vi "m300pmReport.vi"() -> ()   [LabVIEW 2012]
uses:
  <vilib>/addons/database/Auxilliary.llb/DB Tools Cursor Type.ctl
  <vilib>/Utility/NIReport.llb/NI_report.lvclass
  <vilib>/addons/database/Connection.llb/DB Tools Open Connec (Path).vi
  <vilib>/addons/database/Connection.llb/Conn Execute.vi
  <vilib>/addons/database/Recordset.llb/Rec Fetch Recordset Data (R).vi
  <vilib>/addons/database/Recordset.llb/Rec Destroy - Connection.vi
  <vilib>/Utility/NIReport.llb/Append Text Table to Report (wrap).vi
  <vilib>/addons/database/_DB Variant To Data/Database Variant To Data.xnode
  <vilib>/addons/database/NI_Database_API.lvlib
  <vilib>/Utility/NIReport.llb/Excel/NI_Excel.lvclass
  <vilib>/addons/_office/NI_ReportGenerationToolkit.lvlib
  <vilib>/Utility/SMTP/NI_SMTPEmail.lvlib
panel:
  out "error out 2":errorcluster
  out "concatenated string 2":string
  out "error out 4":errorcluster
  in  "MIME content-type (application/octet-stream)":string="application/octet-stream"
  out "error out 3":errorcluster
  out "concatenated string":string
  in  "transposed array":string[][](array[string])
  out "error out":errorcluster
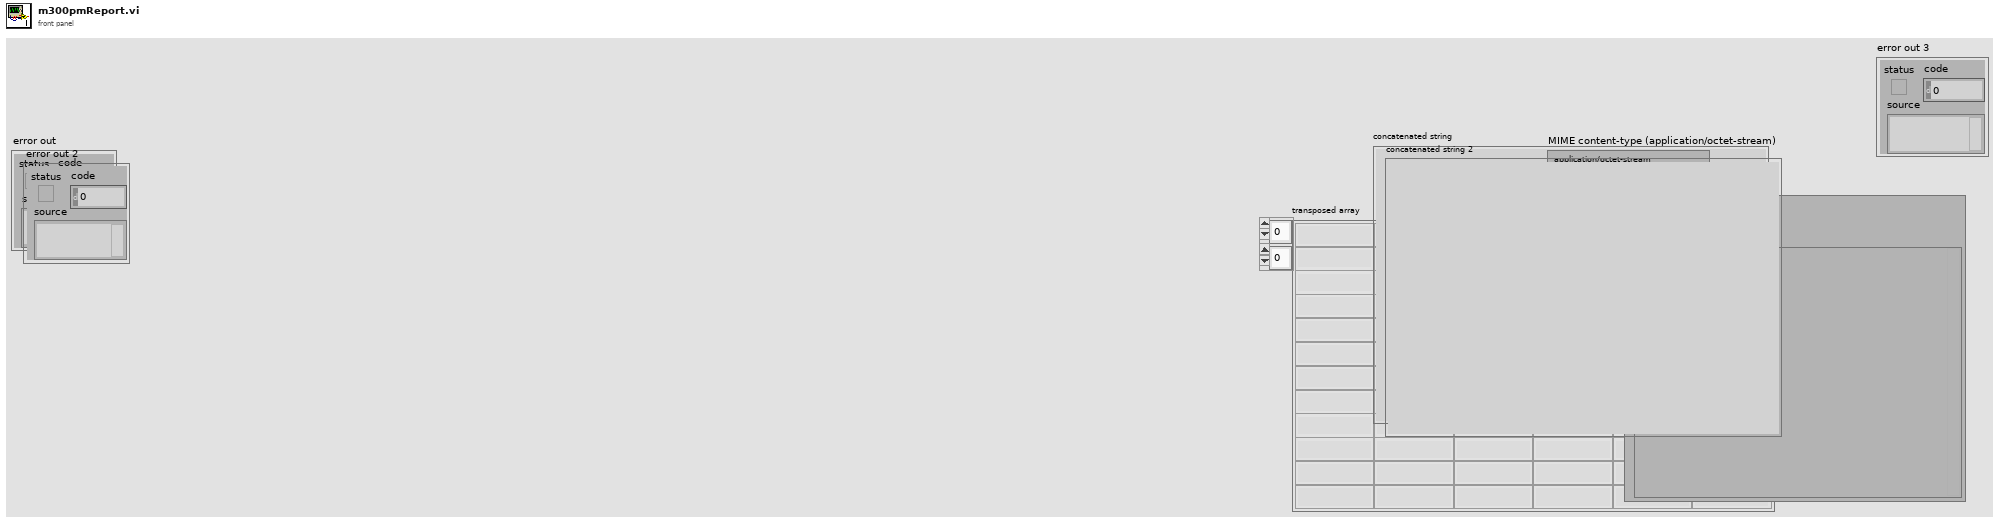
[diagram p1: front panel]
types:
  T1 = enum16{"Standard Report", "HTML", "Word", "Excel"}
  T2 = typedef "NI_Database_API.lvlib/DB Tools Cursor Type.ctl" = enum16{"forward-only", "keyset", "dynamic", "static"}
  T3 = typedef "NI_Database_API.lvlib/Conn ObjectReference.ctl" = refnum<k1>
  T4 = typedef "NI_Database_API.lvlib/Rec ObjectReference.ctl" = refnum<k1>
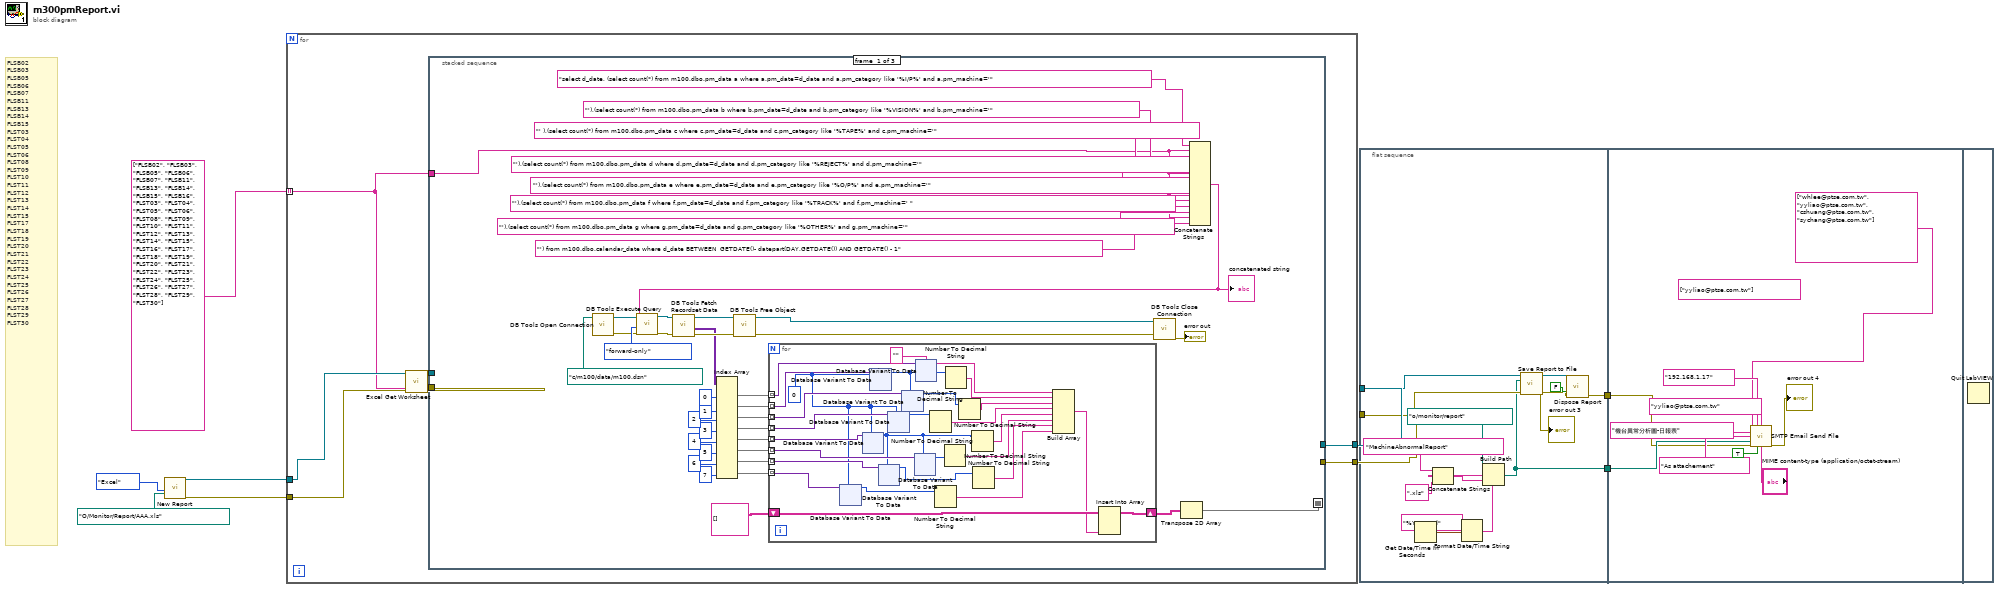
[diagram p0: block diagram]
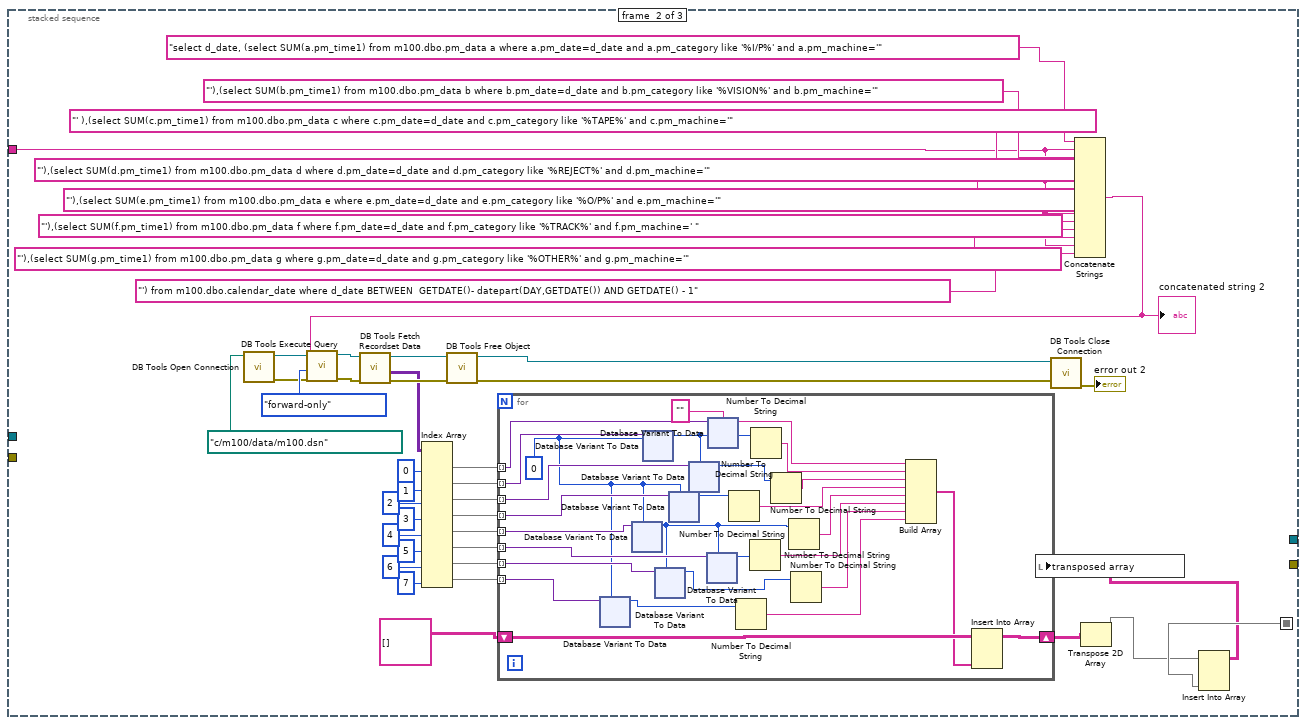
[diagram p2: hidden frame]
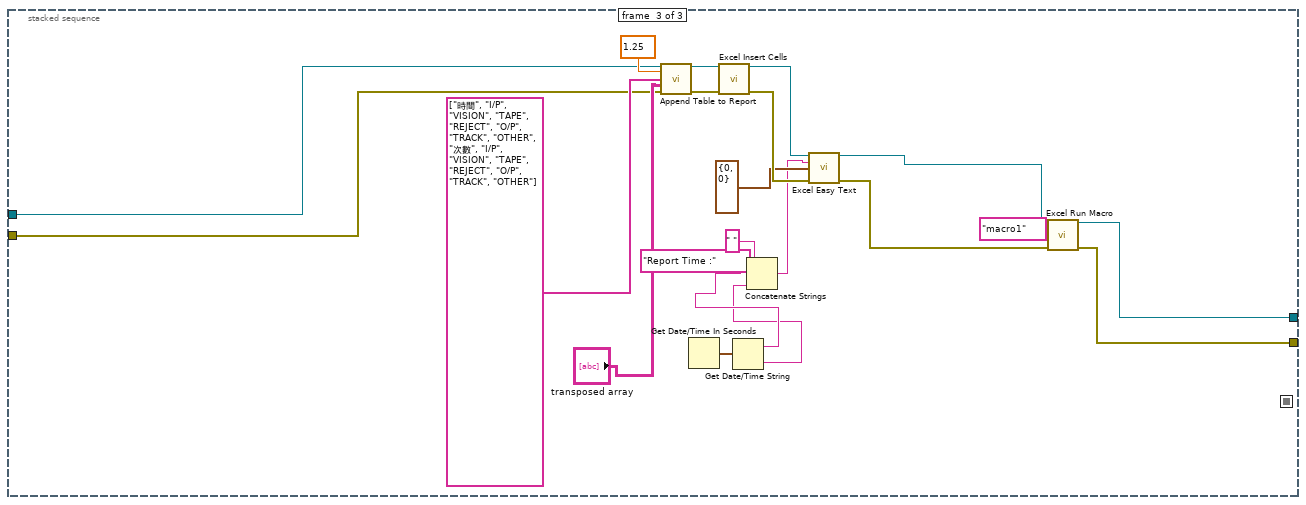
[diagram p3: hidden frame]
diagram:
  # "FLSB02    \nFLSB03    \nFLSB05    \nFLSB06    \nFLSB07    \nFLSB11    \nFLSB13    \nFLSB14    \nFLSB15    \nFLST03    \nFLST04    \nFLST05    \nFLST06    \nFLST08    \nFLST09    \nFLST10    \nFLST11    \nFLST12    \nFLST13    \nFLST14    \nFLST15    \nFLST17    \nFLST18    \nFLST19    \nFLST20    \nFLST21    \nFLST22    \nFLST23    \nFLST24    \nFLST25    \nFLST26    \nFLST27    \nFLST28    \nFLST29    \nFLST30"
  n1 = call <vilib>:"New Report.vi"("report type"=T1."Excel" ("Report Type"), "template (empty)"=path "O:/Monitor/Report/AAA.xls") -> ("report out"=w7:refnum<class "NI_report.lvclass">, "error out"=w6:errorcluster)  [unwired: 12 in]
  n2 = for {
    tunnel: w7 -> [w16]
    tunnel: w6 -> [w15]
    tunnel: string[] ["FLSB02", "FLSB03", "FLSB05", "FLSB06", "FLSB07", "FLSB11", "FLSB13", "FLSB14", "FLSB15", "FLSB16", "FLST03", "FLST04", "FLST05", "FLST06", "FLST08", "FLST09", "FLST10", "FLST11", "FLST12", "FLST13", "FLST14", "FLST15", "FLST16", "FLST17", "FLST18", "FLST19", "FLST20", "FLST21", "FLST22", "FLST23", "FLST24", "FLST25", "FLST26", "FLST27", "FLST28", "FLST29", "FLST30"] -> [w12] mode=indexing
    tunnel: [w11] -> w2
    tunnel: [w10] -> w1
    n3 = call <vilib>:"Excel Get Worksheet.vi"("report in"=w16, "error in (no error)"=w15, "name (\"\")"=w12) -> ("report out"=w14:refnum<class "NI_report.lvclass">, "error out"=w13:errorcluster)  [unwired: 11 in]
    n4 = stacked-sequence {
      seq-local: [w28 _ _] -> [_ w354 _]
      tunnel: w14 -> [_ _ w675]
      tunnel: w13 -> [_ _ w674]
      tunnel: w12 -> [w17 w342 _]
      tunnel: [_ _ w672] -> w11
      tunnel: [_ _ w671] -> w10
      frame #0 {
        n5 = call-poly <vilib>:"DB Tools Open Connection.vi"("connection information"=path "c:/m100/data/m100.dsn") -> ("error out"=w30:errorcluster, "connection reference"=w29:T3)  [unwired: 7 in]
        n6 = Concatenate Strings("select d_date, (select count(*) from m100.dbo.pm_data a where a.pm_date=d_date and a.pm_category like '%I/P%' and a.pm_machine='" ("SQL query"), w17, "'),(select count(*) from m100.dbo.pm_data b where b.pm_date=d_date and b.pm_category like '%VISION%' and b.pm_machine='" ("string"), w17, "' ),(select count(*) from m100.dbo.pm_data c where c.pm_date=d_date and c.pm_category like '%TAPE%' and c.pm_machine='" ("string"), w17, "'),(select count(*) from m100.dbo.pm_data d where d.pm_date=d_date and d.pm_category like '%REJECT%' and d.pm_machine='" ("string"), w17, "'),(select count(*) from m100.dbo.pm_data e where e.pm_date=d_date and e.pm_category like '%O/P%' and e.pm_machine='" ("string"), w17, "'),(select count(*) from m100.dbo.pm_data f where f.pm_date=d_date and f.pm_category like '%TRACK%' and f.pm_machine=' " ("string"), w17, "'),(select count(*) from m100.dbo.pm_data g where g.pm_date=d_date and g.pm_category like '%OTHER%' and g.pm_machine='" ("string"), w17, "') from m100.dbo.calendar_date where d_date BETWEEN  GETDATE()- datepart(DAY,GETDATE()) AND GETDATE() - 1" ("string")) -> (w18:string)
        "concatenated string" <- w18
        n7 = call-poly <vilib>:"DB Tools Execute Query.vi"("error in (no error)"=w30, "cursor type"=DB_Tools_Cursor_Type."forward-only", "SQL query"=w18, "connection reference"=w29) -> ("error out"=w51:errorcluster, "recordset reference"=w53:T4)  [unwired: 4 in]
        n8 = call-poly <vilib>:"DB Tools Fetch Recordset Data.vi"("error in (no error)"=w51, "recordset reference"=w53) -> ("error out"=w50:errorcluster, "recordset data"=w48:variant[][], "recordset reference out"=w52:T4)  [unwired: 3 in]
        n9 = Index Array(array=w48, index (col) #1=0 ("disabled index (col)"), index (col) #2=1 ("index (col)"), index (col) #3=2 ("index (col)"), index (col) #4=3 ("index (col)"), index (col) #5=4 ("index (col)"), index (col) #6=5 ("index (col)"), index (col) #7=6 ("index (col)"), index (col) #8=7 ("index (col)")) -> (element #1=w45:variant[], element #2=w44:variant[], element #3=w36:variant[], element #4=w35:variant[], element #5=w34:variant[], element #6=w33:variant[], element #7=w32:variant[], element #8=w31:variant[])  [unwired: 8 in]
        n10 = call-poly <vilib>:"DB Tools Free Object.vi"("error in (no error)"=w50, "recordset reference"=w52) -> ("error out"=w54:errorcluster, "connection reference"=w55:T3)  [unwired: 8 in]
        n11 = for {
          tunnel: w45 -> [w84] mode=indexing
          tunnel: w44 -> [w85] mode=indexing
          shift-right: [w80] -> w27
          shift-left: string[][] [] ("array") -> [w79]
          tunnel: w36 -> [w77] mode=indexing
          tunnel: w35 -> [w76] mode=indexing
          tunnel: w34 -> [w75] mode=indexing
          tunnel: w33 -> [w74] mode=indexing
          tunnel: w32 -> [w71] mode=indexing
          tunnel: w31 -> [w68] mode=indexing
          w67 = 0
          n12 = xnode "Database Variant To Data"("database variant"=w68, "type"=w67) -> ("data"=w66:i32)  [unwired: 1 in, 1 out]
          n13 = xnode "Database Variant To Data"("database variant"=w75, "type"=w67) -> ("data"=w69:i32)  [unwired: 1 in, 1 out]
          n14 = xnode "Database Variant To Data"("database variant"=w85, "type"=w67) -> ("data"=w65:i32)  [unwired: 1 in, 1 out]
          n15 = xnode "Database Variant To Data"("database variant"=w71, "type"=w69) -> ("data"=w70:i32)  [unwired: 1 in, 1 out]
          n16 = xnode "Database Variant To Data"("database variant"=w76, "type"=w67) -> ("data"=w73:i32)  [unwired: 1 in, 1 out]
          n17 = xnode "Database Variant To Data"("database variant"=w77, "type"=w65) -> ("data"=w64:i32)  [unwired: 1 in, 1 out]
          n18 = xnode "Database Variant To Data"("database variant"=w74, "type"=w69) -> ("data"=w72:i32)  [unwired: 1 in, 1 out]
          n19 = xnode "Database Variant To Data"("database variant"=w84, "type"="") -> ("data"=w82:string)  [unwired: 1 in, 1 out]
          n20 = Number To Decimal String(number=w73) -> (decimal integer string=w59:string)  [unwired: 1 in]
          n21 = Number To Decimal String(number=w66) -> (decimal integer string=w63:string)  [unwired: 1 in]
          n22 = Number To Decimal String(number=w72) -> (decimal integer string=w61:string)  [unwired: 1 in]
          n23 = Number To Decimal String(number=w65) -> (decimal integer string=w81:string)  [unwired: 1 in]
          n24 = Number To Decimal String(number=w64) -> (decimal integer string=w58:string)  [unwired: 1 in]
          n25 = Number To Decimal String(number=w69) -> (decimal integer string=w60:string)  [unwired: 1 in]
          n26 = Number To Decimal String(number=w70) -> (decimal integer string=w62:string)  [unwired: 1 in]
          n27 = Build Array(w82, w81, w58, w59, w60, w61, w62, w63) -> (w78:string[])
          n28 = Insert Into Array(array=w79, new element=w78) -> (w80:string[][])  [unwired: 2 in]
        }
        n29 = call <vilib>:"DB Tools Close Connection.vi"("error in (no error)"=w54, "connection reference"=w55) -> ("error out"=→"error out":errorcluster)  [unwired: 5 in]
        n30 = Transpose 2D Array(2D array=w27) -> (transposed array=w28:string[][])
      }
      frame #1 {
        n31 = call-poly <vilib>:"DB Tools Open Connection.vi"("connection information"=path "c:/m100/data/m100.dsn") -> ("error out"=w358:errorcluster, "connection reference"=w357:T3)  [unwired: 7 in]
        n32 = Concatenate Strings("select d_date, (select SUM(a.pm_time1) from m100.dbo.pm_data a where a.pm_date=d_date and a.pm_category like '%I/P%' and a.pm_machine='" ("SQL query"), w342, "'),(select SUM(b.pm_time1) from m100.dbo.pm_data b where b.pm_date=d_date and b.pm_category like '%VISION%' and b.pm_machine='" ("string"), w342, "' ),(select SUM(c.pm_time1) from m100.dbo.pm_data c where c.pm_date=d_date and c.pm_category like '%TAPE%' and c.pm_machine='" ("string"), w342, "'),(select SUM(d.pm_time1) from m100.dbo.pm_data d where d.pm_date=d_date and d.pm_category like '%REJECT%' and d.pm_machine='" ("string"), w342, "'),(select SUM(e.pm_time1) from m100.dbo.pm_data e where e.pm_date=d_date and e.pm_category like '%O/P%' and e.pm_machine='" ("string"), w342, "'),(select SUM(f.pm_time1) from m100.dbo.pm_data f where f.pm_date=d_date and f.pm_category like '%TRACK%' and f.pm_machine=' " ("string"), w342, "'),(select SUM(g.pm_time1) from m100.dbo.pm_data g where g.pm_date=d_date and g.pm_category like '%OTHER%' and g.pm_machine='" ("string"), w342, "') from m100.dbo.calendar_date where d_date BETWEEN  GETDATE()- datepart(DAY,GETDATE()) AND GETDATE() - 1" ("string")) -> (w343:string)
        "concatenated string 2" <- w343
        n33 = call-poly <vilib>:"DB Tools Execute Query.vi"("error in (no error)"=w358, "cursor type"=DB_Tools_Cursor_Type."forward-only", "SQL query"=w343, "connection reference"=w357) -> ("error out"=w378:errorcluster, "recordset reference"=w380:T4)  [unwired: 4 in]
        n34 = call-poly <vilib>:"DB Tools Fetch Recordset Data.vi"("error in (no error)"=w378, "recordset reference"=w380) -> ("error out"=w377:errorcluster, "recordset data"=w375:variant[][], "recordset reference out"=w379:T4)  [unwired: 3 in]
        n35 = Index Array(array=w375, index (col) #1=0 ("disabled index (col)"), index (col) #2=1 ("index (col)"), index (col) #3=2 ("index (col)"), index (col) #4=3 ("index (col)"), index (col) #5=4 ("index (col)"), index (col) #6=5 ("index (col)"), index (col) #7=6 ("index (col)"), index (col) #8=7 ("index (col)")) -> (element #1=w372:variant[], element #2=w371:variant[], element #3=w364:variant[], element #4=w363:variant[], element #5=w362:variant[], element #6=w361:variant[], element #7=w360:variant[], element #8=w359:variant[])  [unwired: 8 in]
        n36 = call-poly <vilib>:"DB Tools Free Object.vi"("error in (no error)"=w377, "recordset reference"=w379) -> ("error out"=w381:errorcluster, "connection reference"=w382:T3)  [unwired: 8 in]
        n37 = for {
          tunnel: w372 -> [w411] mode=indexing
          tunnel: w371 -> [w412] mode=indexing
          shift-right: [w407] -> w356
          shift-left: string[][] [] ("array") -> [w406]
          tunnel: w364 -> [w404] mode=indexing
          tunnel: w363 -> [w403] mode=indexing
          tunnel: w362 -> [w402] mode=indexing
          tunnel: w361 -> [w401] mode=indexing
          tunnel: w360 -> [w398] mode=indexing
          tunnel: w359 -> [w395] mode=indexing
          w394 = 0
          n38 = xnode "Database Variant To Data"("database variant"=w395, "type"=w394) -> ("data"=w393:i32)  [unwired: 1 in, 1 out]
          n39 = xnode "Database Variant To Data"("database variant"=w402, "type"=w394) -> ("data"=w396:i32)  [unwired: 1 in, 1 out]
          n40 = xnode "Database Variant To Data"("database variant"=w412, "type"=w394) -> ("data"=w392:i32)  [unwired: 1 in, 1 out]
          n41 = xnode "Database Variant To Data"("database variant"=w398, "type"=w396) -> ("data"=w397:i32)  [unwired: 1 in, 1 out]
          n42 = xnode "Database Variant To Data"("database variant"=w403, "type"=w394) -> ("data"=w400:i32)  [unwired: 1 in, 1 out]
          n43 = xnode "Database Variant To Data"("database variant"=w404, "type"=w392) -> ("data"=w391:i32)  [unwired: 1 in, 1 out]
          n44 = xnode "Database Variant To Data"("database variant"=w401, "type"=w396) -> ("data"=w399:i32)  [unwired: 1 in, 1 out]
          n45 = xnode "Database Variant To Data"("database variant"=w411, "type"="") -> ("data"=w409:string)  [unwired: 1 in, 1 out]
          n46 = Number To Decimal String(number=w400) -> (decimal integer string=w386:string)  [unwired: 1 in]
          n47 = Number To Decimal String(number=w393) -> (decimal integer string=w390:string)  [unwired: 1 in]
          n48 = Number To Decimal String(number=w399) -> (decimal integer string=w388:string)  [unwired: 1 in]
          n49 = Number To Decimal String(number=w392) -> (decimal integer string=w408:string)  [unwired: 1 in]
          n50 = Number To Decimal String(number=w391) -> (decimal integer string=w385:string)  [unwired: 1 in]
          n51 = Number To Decimal String(number=w396) -> (decimal integer string=w387:string)  [unwired: 1 in]
          n52 = Number To Decimal String(number=w397) -> (decimal integer string=w389:string)  [unwired: 1 in]
          n53 = Build Array(w409, w408, w385, w386, w387, w388, w389, w390) -> (w405:string[])
          n54 = Insert Into Array(array=w406, new element=w405) -> (w407:string[][])  [unwired: 2 in]
        }
        n55 = call <vilib>:"DB Tools Close Connection.vi"("error in (no error)"=w381, "connection reference"=w382) -> ("error out"=→"error out 2":errorcluster)  [unwired: 5 in]
        n56 = Transpose 2D Array(2D array=w356) -> (transposed array=w353:string[][])
        n57 = Insert Into Array(array=w353, new element=w354) -> (w352:string[][])  [unwired: 2 in]
        n58 = local write "transposed array"(w352) -> ()
      }
      frame #2 {
        n59 = call-poly <vilib>:"Append Table to Report.vi"("report in"=w675, "column width (1)"=1.25, "row headers"=string[] ["時間", "I/P", "VISION", "TAPE", "REJECT", "O/P", "TRACK", "OTHER", "次數", "I/P", "VISION", "TAPE", "REJECT", "O/P", "TRACK", "OTHER"], "text data"="transposed array", "error in (no error)"=w674) -> ("report out"=w688:refnum<class "NI_report.lvclass">, "error out"=w687:errorcluster)  [unwired: 7 in, 2 out]
        n60 = Get Date/Time In Seconds() -> (seconds since 1Jan1904=w682:timestamp)
        n61 = call <vilib>:"Excel Insert Cells.vi"("report in"=w688, "error in (no error)"=w687) -> ("report out"=w686:refnum<class "NI_report.lvclass">, "error out"=w685:errorcluster)  [unwired: 12 in]
        n62 = Get Date/Time String(seconds (now)=w682) -> (date string=w681:string, time string=w679:string)  [unwired: 2 in]
        n63 = Concatenate Strings("Report Time :" ("string"), w681, " " ("string"), w679) -> (w678:string)
        n64 = call <vilib>:"Excel Easy Text.vi"("report in"=w686, "text"=w678, "start (-1, -1)"=cluster{"row":i32, "column":i32} {"row"=0, "column"=0} ("end (-1, -1)"), "error in (no error)"=w685) -> ("report out"=w670:refnum<class "NI_report.lvclass">, "error out"=w669:errorcluster)  [unwired: 7 in, 3 out]
        n65 = call <vilib>:"Excel Run Macro.vi"("report in"=w670, "macro name"="macro1", "error in (no error)"=w669) -> ("report out"=w672:refnum<class "NI_report.lvclass">, "error out"=w671:errorcluster)  [unwired: 10 in, 1 out]
      }
    }
  }
  n66 = flat-sequence {
    tunnel: w2 -> [w699]
    tunnel: w1 -> [w698]
    tunnel: [w692] -> w4
    tunnel: [w691] -> w3
    tunnel: w4 -> [w705]
    tunnel: w3 -> [w706]
    frame #0 {
      n67 = Get Date/Time In Seconds() -> (seconds since 1Jan1904=w695:timestamp)
      n68 = Format Date/Time String(time format string (%c)="%Y%m%d", seconds (now)=w695) -> (date/time string=w693:string)  [unwired: 1 in]
      n69 = Concatenate Strings("MachineAbnormalReport" ("string"), w693, ".xls" ("string")) -> (w700:string)
      n70 = Build Path(base path=path "o:/monitor/report", name or relative path=w700) -> (appended path=w691:path)
      n71 = call-dynamic "Save Report to File.vi"("report in"=w699, "report file path"=w691, "error in (no error)"=w698) -> ("report out"=w702:refnum<class "NI_report.lvclass">, "error out"=w701:errorcluster)  [unwired: 11 in]
      "error out 3" <- w701
      n72 = call-dynamic "Dispose Report.vi"("report in"=w702, "save changes? (F)"=FALSE, "error in (no error)"=w701) -> ("error out"=w692:errorcluster)  [unwired: 12 in]
    }
    frame #1 {
      (unwired) string[] ["yyliao@ptse.com.tw"] ("recipients")
      n73 = call <vilib>:"SMTP Email Send File.vi"("recipients"=string[] ["whlee@ptse.com.tw", "yyliao@ptse.com.tw", "cshuang@ptse.com.tw", "sychang@ptse.com.tw"], "mail server"="192.168.1.17", "return address"="yyliao@ptse.com.tw", "subject ([No Subject])"="機台異常分析圖-日報表", "message"="As attachement", "file path"=w706, "error in (no error)"=w705, "binary? (F)"=TRUE, "MIME content-type (application/octet-stream)"="MIME content-type (application/octet-stream)") -> ("error out"=→"error out 4":errorcluster)  [unwired: 5 in, 1 out]
    }
    frame #2 {
      n74 = Quit LabVIEW() -> ()  [unwired: 1 in]
    }
  }
